vi "Get File Type Icon Image.vi"(8 "error in (no error)":errorcluster, 11 "path":path) -> (0 "error out":errorcluster, 3 "image data":T1)   [LabVIEW 2014, in "NI_FileType.lvlib"]
doc: "Returns TRUE if this file could be loaded with the Open VI Reference function. It includes VIs, Polymorphic VIs, Controls, Templates, and Globals."
uses:
  NI_FileType.lvlib
  imagedata.ctl
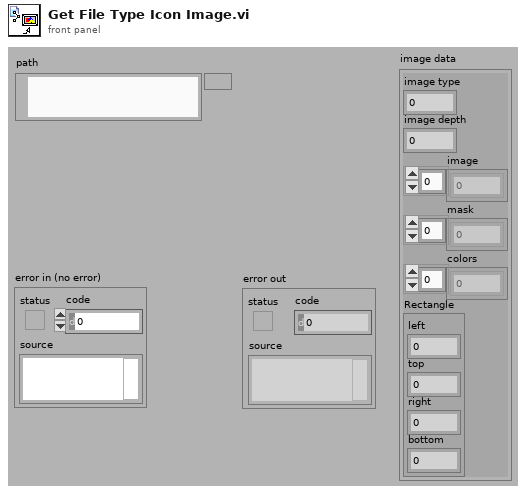
[diagram p1: front panel]
types:
  T1 = typedef "imagedata.ctl" = cluster{"image type":i32, "image depth":i32, "image":u8[], "mask":u8[], "colors":u32[], "Rectangle":cluster{"left":i16, "top":i16, "right":i16, "bottom":i16}}
  T2 = typedef "NI_FileType.lvlib/FT_FileTypes.ctl" = enum32{"Invalid file/path", "Unknown type", "Instrument", "Control", "Polymorphic VI", "Project", "Library", "LVClass", "XControl", "XNode", "CIN", "Run-time menu", "Palette menu", "LLB", "Shortcut", "Directory", "Class Private Data Control", "Statechart", "MathScript .m file", "Ladder Diagram", "LVLibp"}
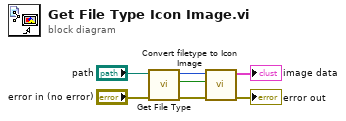
[diagram p0: block diagram]
diagram:
  n1 = call "Get File Type.vi"("error in (no error)"="error in (no error)", "path"="path") -> ("error out"=w3:errorcluster, "is template?"=w1:bool, "file type"=w5:T2)  [unwired: 7 in]
  n2 = call "Convert filetype to Icon Image.vi"("error in (no error)"=w3, "is template?"=w1, "file type"=w5) -> ("error out"=→"error out":errorcluster, "image data"=→"image data":T1)  [unwired: 7 in]
